vi "Initialise Sound And Music.vi"(8 "error in (no error)":errorcluster, 11 "Main Controller Actor in":refnum<class "Main Controller Actor.lvclass">) -> (0 "error out":errorcluster, 3 "Main Controller Actor out":refnum<class "Main Controller Actor.lvclass">)   [LabVIEW 2015, in "Main Controller Actor.lvclass"]
uses:
  Main Controller Actor.lvclass
  <vilib>/Utility/file.llb/Application Directory.vi
  LabBASSMOD2/LabBassMOD2.lvlib
  LabSDL2/Source/Libraries/LibSDL2_Mixer Wrapper/LibSDL2_Mixer.lvlib
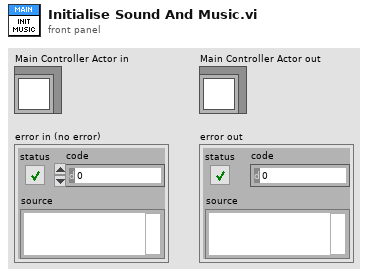
[diagram p1: front panel]
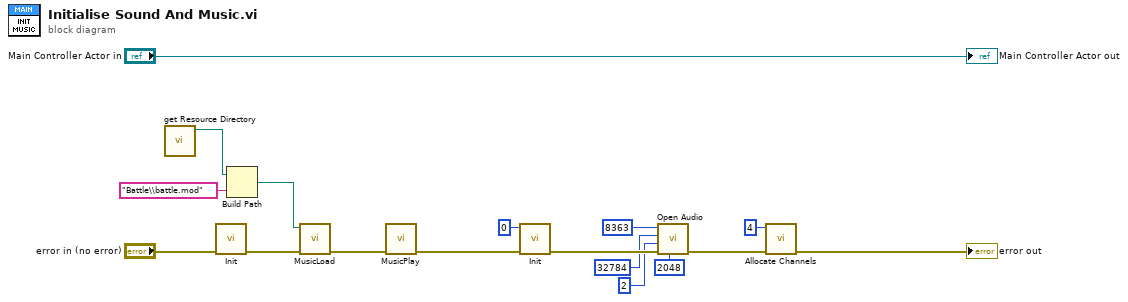
[diagram p0: block diagram]
diagram:
  n1 = call "get Resource Directory.vi"() -> ("Resource Directory"=w13:path)  [unwired: 11 in]
  n2 = call "Init.vi"("error in (no error)"="error in (no error)") -> ("error out"=w11:errorcluster)  [unwired: 9 in, 1 out]
  n3 = Build Path(base path=w13, name or relative path="Battle\\battle.mod") -> (appended path=w14:path)
  n4 = call "MusicLoad.vi"("error in (no error)"=w11, "path"=w14) -> ("error out"=w15:errorcluster)  [unwired: 9 in]
  n5 = call "MusicPlay.vi"("error in (no error)"=w15) -> ("error out"=w2:errorcluster)  [unwired: 10 in]
  n6 = call "Init.vi"("error in"=w2, "Flags"=0) -> ("error out"=w10:errorcluster)  [unwired: 8 in, 1 out]
  n7 = call "Open Audio.vi"("Chunksize"=2048, "error in"=w10, "Channels"=2, "Format"=u16 32784, "Frequency"=8363) -> ("error out"=w4:errorcluster)  [unwired: 5 in, 1 out]
  n8 = call "Allocate Channels.vi"("error in"=w4, "Num Channels"=4) -> ("error out"=→"error out":errorcluster)  [unwired: 8 in, 1 out]
  "Main Controller Actor out" <- "Main Controller Actor in"
